vi "mongo_run_command.vi"(9 "db":string, 10 "conn":T2, 11 "cmd in":T1) -> (0 "result":errorcluster, 2 "out":T1, 3 "cmd out":T1)   [LabVIEW 2013]
uses:
  bson.ctl
  mongo.ctl
  bson_shared_empty.vi
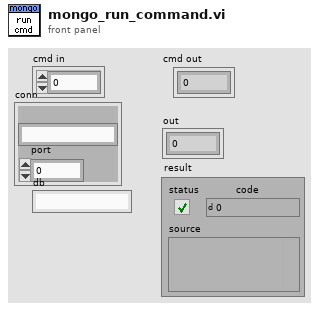
[diagram p1: front panel]
types:
  T1 = typedef "bson.ctl" = cluster{i32}
  T2 = typedef "mongo.ctl" = cluster{"host":string, "port":i32}
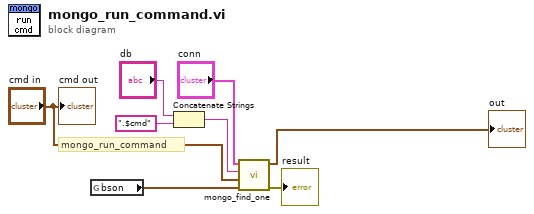
[diagram p0: block diagram]
diagram:
  # "mongo_run_command"
  n1 = global read "bson_shared_empty.vi" "bson"() -> (w3:T1)
  n2 = Concatenate Strings("db", ".$cmd" ("string")) -> (w5:string)
  n3 = call "mongo_find_one.vi"("fields"=w3, "query"="cmd in", "ns"=w5, "mongo"="conn") -> ("error out"=→"result":errorcluster, "out"=→"out":T1)  [unwired: 6 in]
  "cmd out" <- "cmd in"
